vi "ma_Trap Fgen Parameter Errors.vi"(6 "Sampling info":cluster{"Fs":dbl, "#s":i32}={"Fs"=1000.0, "#s"=1000} {"Fs" format="%0.2f"}, 8 "error in (no error)":errorcluster, 10 "frequency":dbl format="%0.2p") -> (0 "error out":errorcluster)   [LabVIEW 2020, in "NI_MABase.lvlib"]
uses:
  NI_MABase.lvlib
panel:
  in  "freq error message":string="frequency must be <= sampling rate/2"
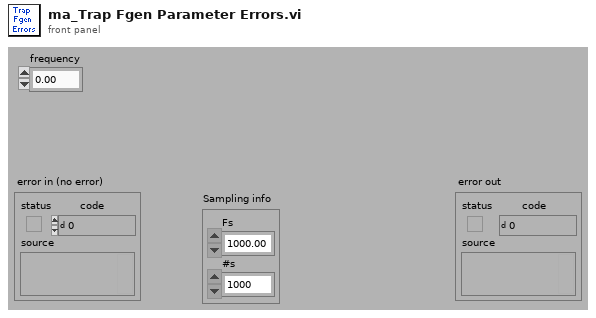
[diagram p1: front panel]
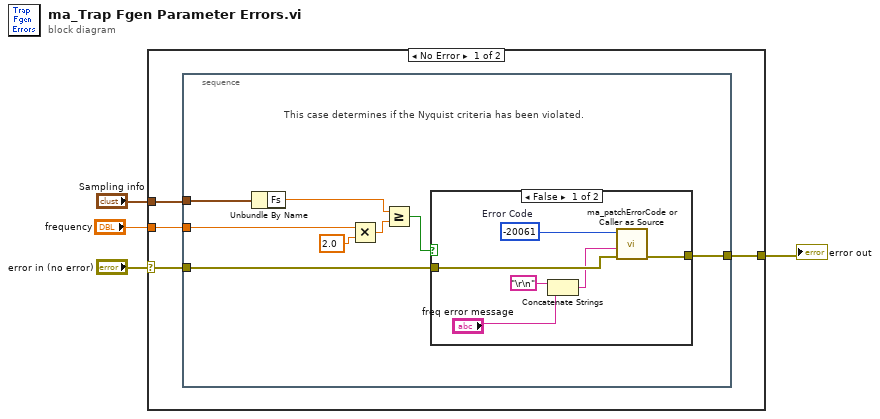
[diagram p0: block diagram]
diagram:
  n1 = case shown="No Error" "error in (no error)" {
    selector: "error in (no error)" -> [w6 w24]
    tunnel: [w5 w24] -> w4
    tunnel: "Sampling info" -> [w8 _]
    tunnel: "frequency" -> [w7 _]
    frame No Error {
      n2 = stacked-sequence {
        tunnel: w8 -> [w12]
        tunnel: [w11] -> w5
        tunnel: w6 -> [w10]
        tunnel: w7 -> [w9]
        frame #0 {
          # "This case determines if the Nyquist criteria has been violated."
          n3 = Unbundle By Name(w12) -> ("Fs"=w14:dbl)
          n4 = Multiply(x=w9, y=2.0) -> (x*y=w15:dbl)
          n5 = Greater Or Equal?(x=w14, y=w15) -> (x >= y?=w16:bool)
          n6 = case shown="False" w16 {
            tunnel: w10 -> [w21 w23]
            tunnel: [w20 w23] -> w11
            frame False {
              w22 = -20061  # Error Code
              n7 = Concatenate Strings("\r\n", "freq error message") -> (w17:string)
              n8 = call "ma_patchErrorCode or Caller as Source.vi"("error in (no error)"=w21, "string to append to source"=w17, "error code"=w22) -> ("error out"=w20:errorcluster)  [unwired: 8 in]
            }
            frame True {
            }
          }
        }
      }
    }
    frame Error {
    }
  }
  "error out" <- w4
